vi "Decimal point.vi"() -> ()   [LabVIEW 2017]
panel:
  out "number":dbl
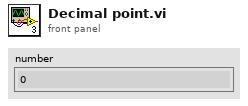
[diagram p1: front panel]
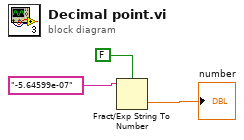
[diagram p0: block diagram]
diagram:
  n1 = Fract/Exp String To Number(use system decimal point (T)=FALSE, string="-5.64599e-07") -> (number=→"number":dbl)  [unwired: 2 in, 1 out]
